vi "Read Log_OccupancyGrid.vi"(8 "error in (no error)":errorcluster, 11 "Probabilistic_OccupancyGrid in":refnum<class "Probabilistic_OccupancyGrid.lvclass">) -> (0 "error out":errorcluster, 2 "Log_OccupancyGrid":dbl[][](array[numeric]), 3 "Probabilistic_OccupancyGrid out":refnum<class "Probabilistic_OccupancyGrid.lvclass">)   [LabVIEW 2017, in "Probabilistic_OccupancyGrid.lvclass"]
uses:
  Probabilistic_OccupancyGrid.lvclass
  Probabilistic_OccupancyGrid.lvclass/Probabilistic_OccupancyGrid.ctl
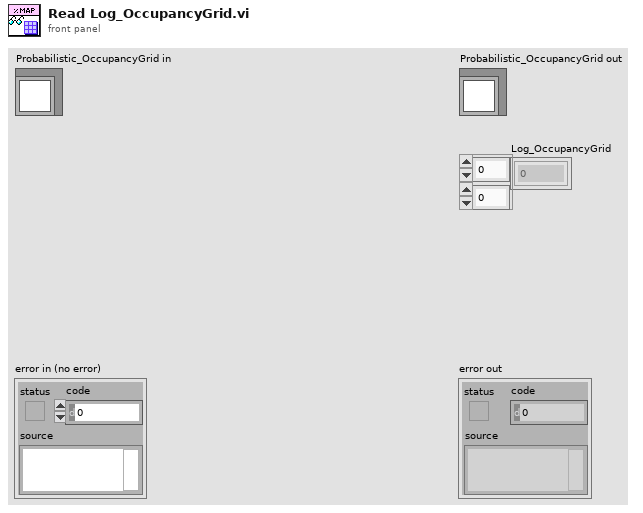
[diagram p1: front panel]
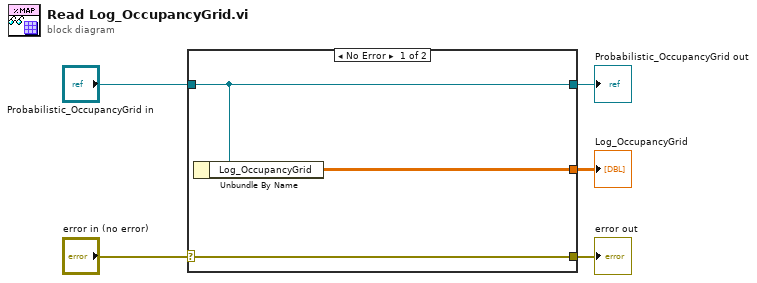
[diagram p0: block diagram]
diagram:
  n1 = case shown="No Error" "error in (no error)" {
    selector: "error in (no error)" -> [w8 w9]
    tunnel: [w8 w9] -> w4
    tunnel: [w7 w10] -> w2
    tunnel: "Probabilistic_OccupancyGrid in" -> [w7 w10]
    tunnel: [w6 _] -> w1
    frame No Error {
      n2 = Unbundle By Name(w7) -> ("Log_OccupancyGrid"=w6:dbl[][])
    }
    frame Error {
    }
  }
  "error out" <- w4
  "Probabilistic_OccupancyGrid out" <- w2
  "Log_OccupancyGrid" <- w1
